vi "UI Laser Page.vi"(8 "error in":errorcluster) -> (0 "error out":errorcluster)   [LabVIEW 2019, in "UIs.lvlib"]
uses:
  UIs.lvlib
  <vilib>/Utility/miscctls.llb/LVPointTypeDef.ctl
  Camera/Andor/Andor.lvlib
  Laser/Coherent/Coherent.lvlib
  Motion/Allmotion/Allmotion.lvlib
  Image/Image.lvlib
  Controller/Controller.lvlib
  Initialize/Initialize.lvlib
panel:
  in  "Align Laser":bool
  in  "Search Focus":bool
  in  "Back":bool
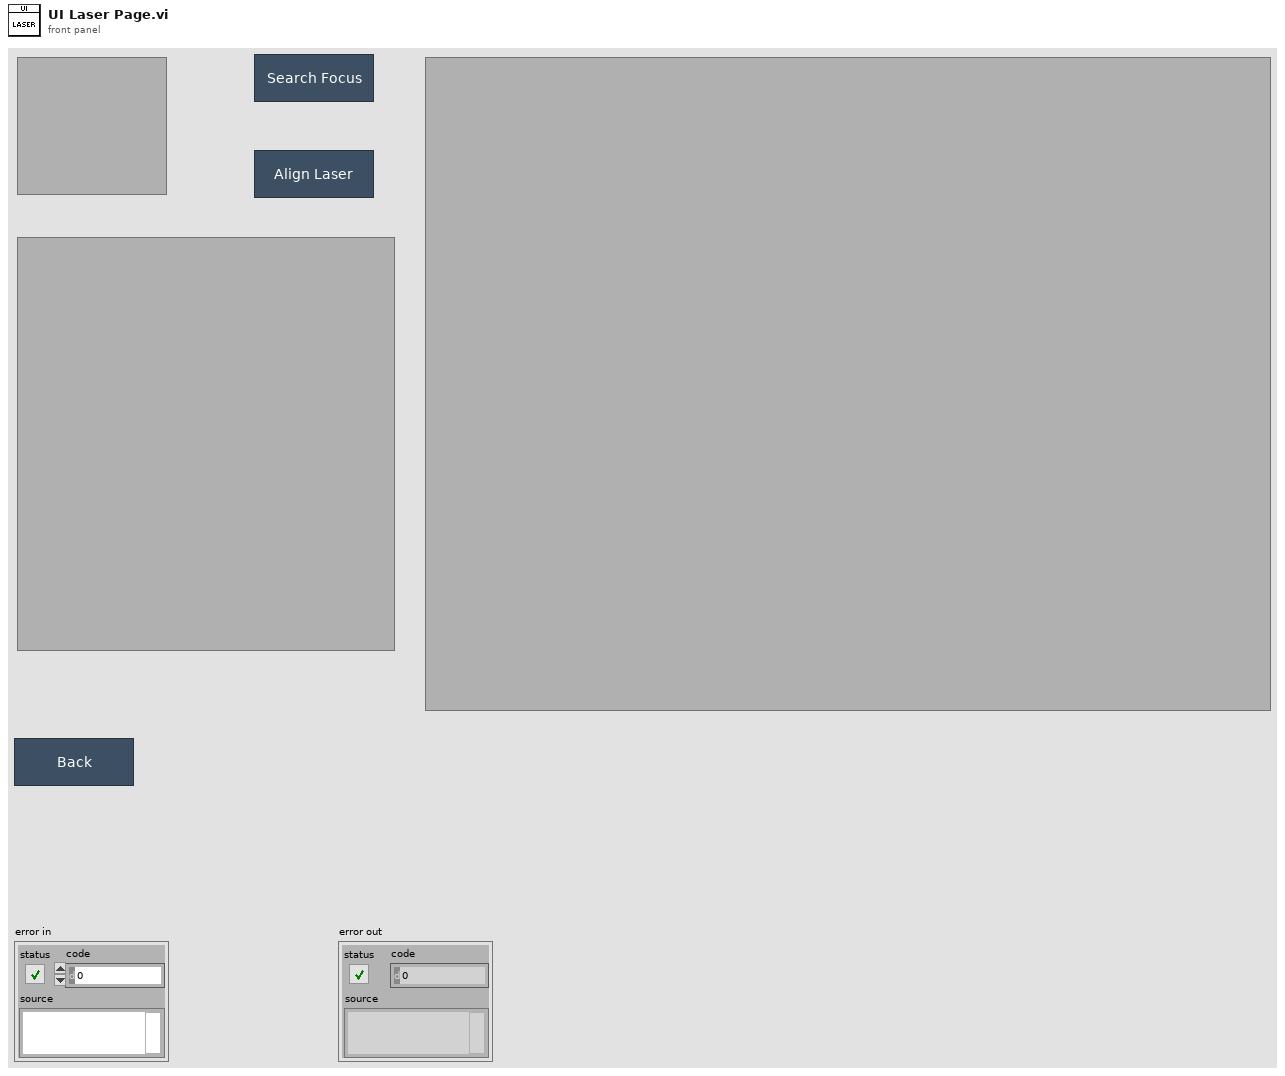
[diagram p1: front panel]
types:
  T1 = typedef "LVPointTypeDef.ctl" = cluster{"Horizontal":i16, "Vertical":i16}
  T2 = typedef "Allmotion.lvlib/SEQ Data.ctl" = cluster{"Position":i32[], "Arrived?":bool, "VISA name":refnum<visa-resource-name>, "Initialize Done?":bool, "State":string, "VI Refnum":refnum<vi>, "Dichroic Position":string[]}
  T3 = typedef "Andor.lvlib/SEQ Data.ctl" = cluster{"Initialize Sucess?":bool, "Image Ref":T4, "VI Refnum":refnum<vi>}
  T4 = typedef "IMAQ Image.ctl" = refnum<image>
  T5 = typedef "Coherent.lvlib/SEQ Data.ctl" = cluster{"Initialize Success?":bool, "VI Refnum":refnum<vi>}
  T6 = typedef "Initialize.lvlib/SEQ Data.ctl" = cluster{"Folder Path":path}
  T7 = typedef "Image.lvlib/SEQ Data.ctl" = cluster{"Acquire Done?":bool, "Focus Done?":bool, "Align Done?":bool, "No Position Match?":bool, "Best Wheel Position":string, "Match Done?":bool, "Match Score":dbl, "Focus Score":dbl, "Match Position":cluster{"x":sgl, "y":sgl}, "Flower Position":i32[]}
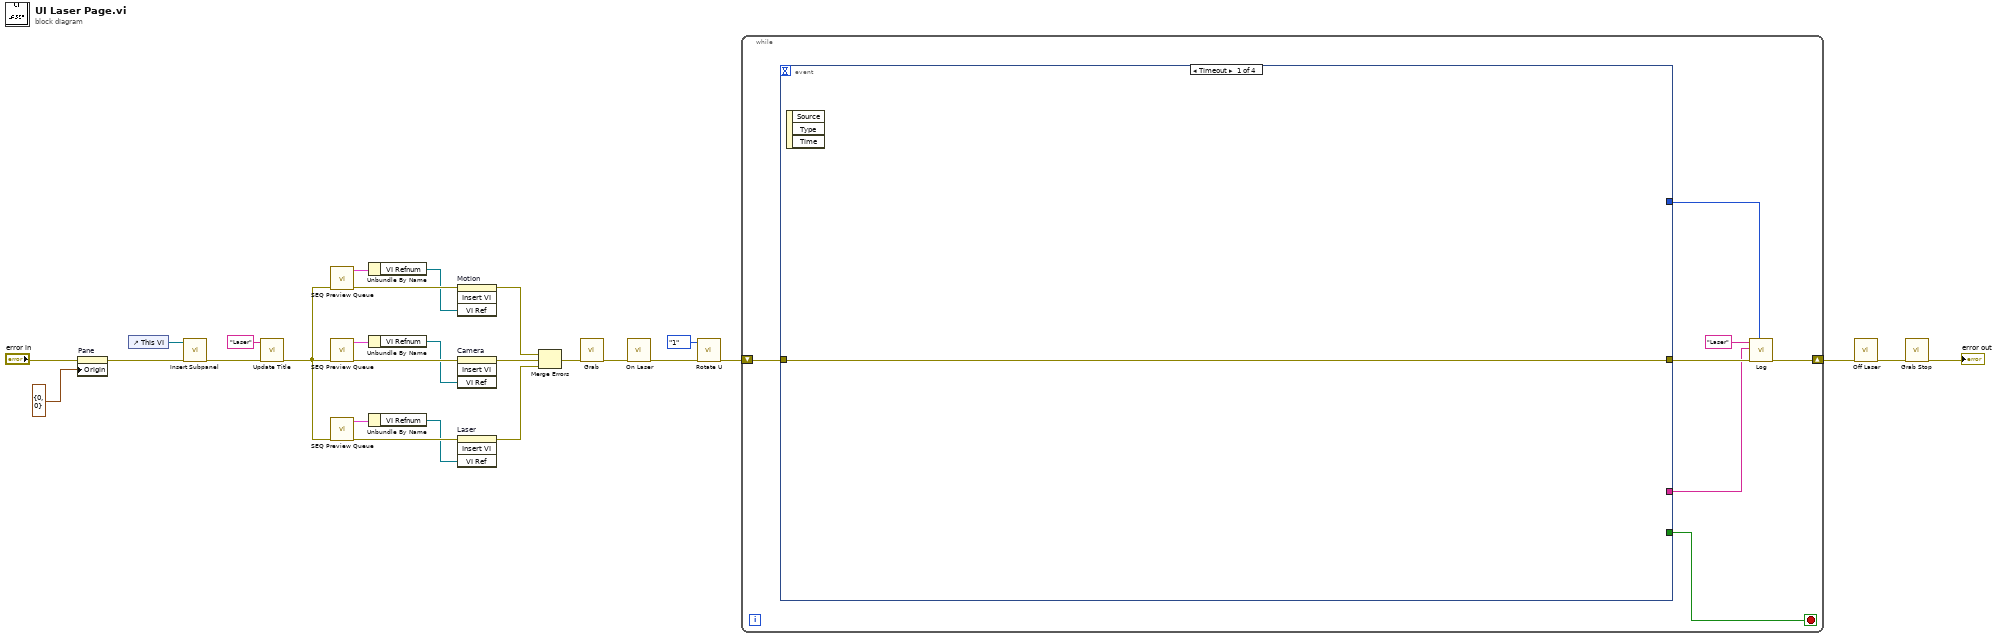
[diagram p0: block diagram]
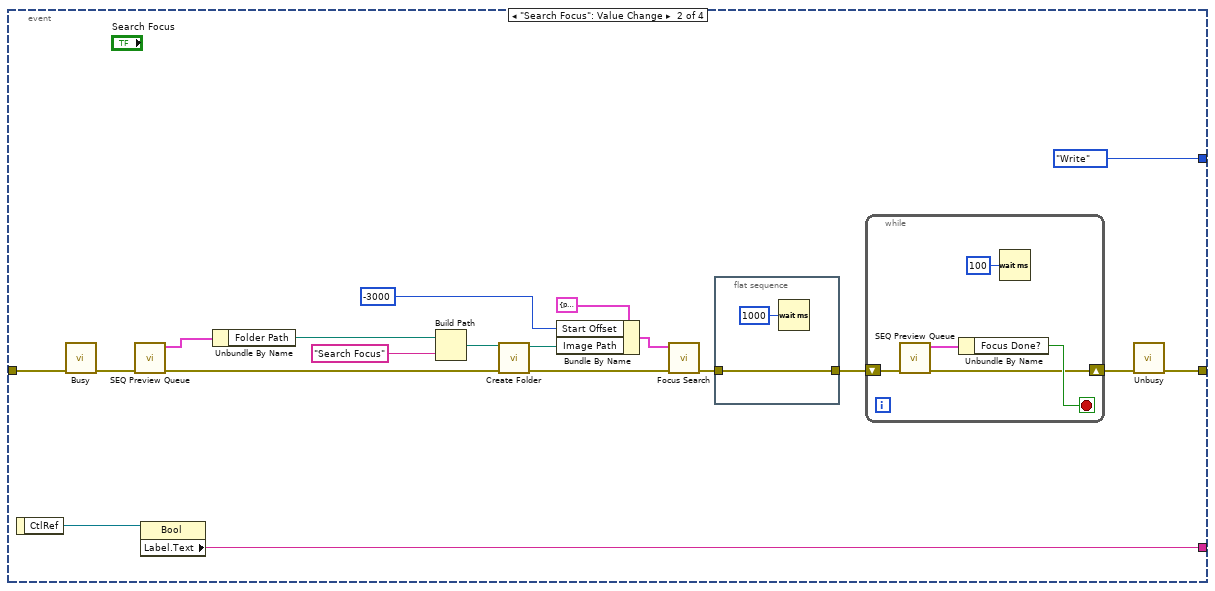
[diagram p2: hidden frame]
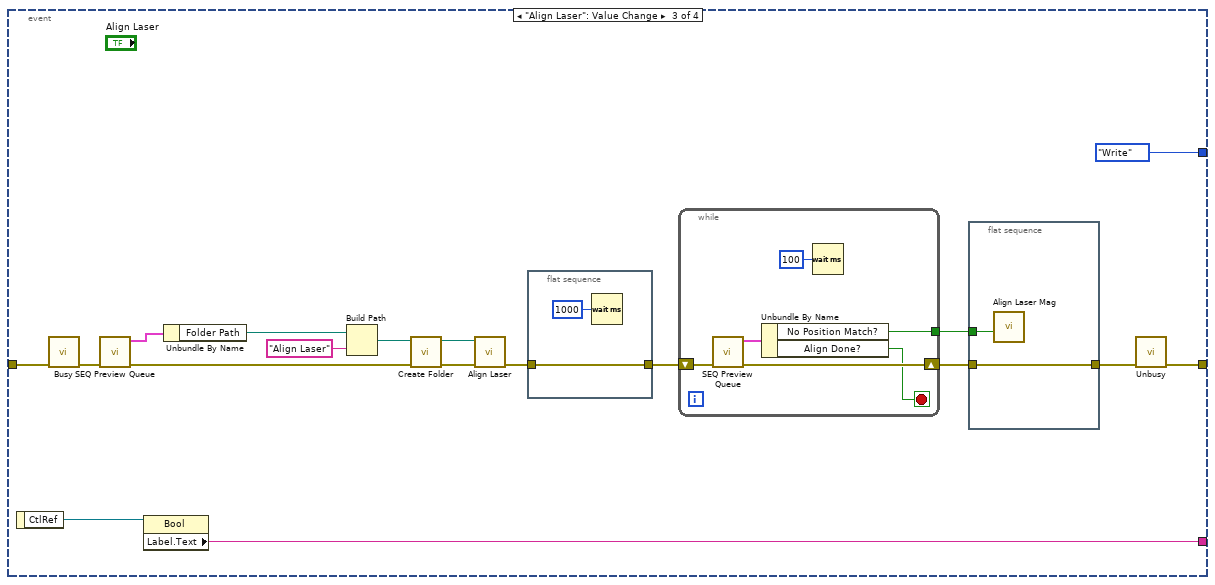
[diagram p3: hidden frame]
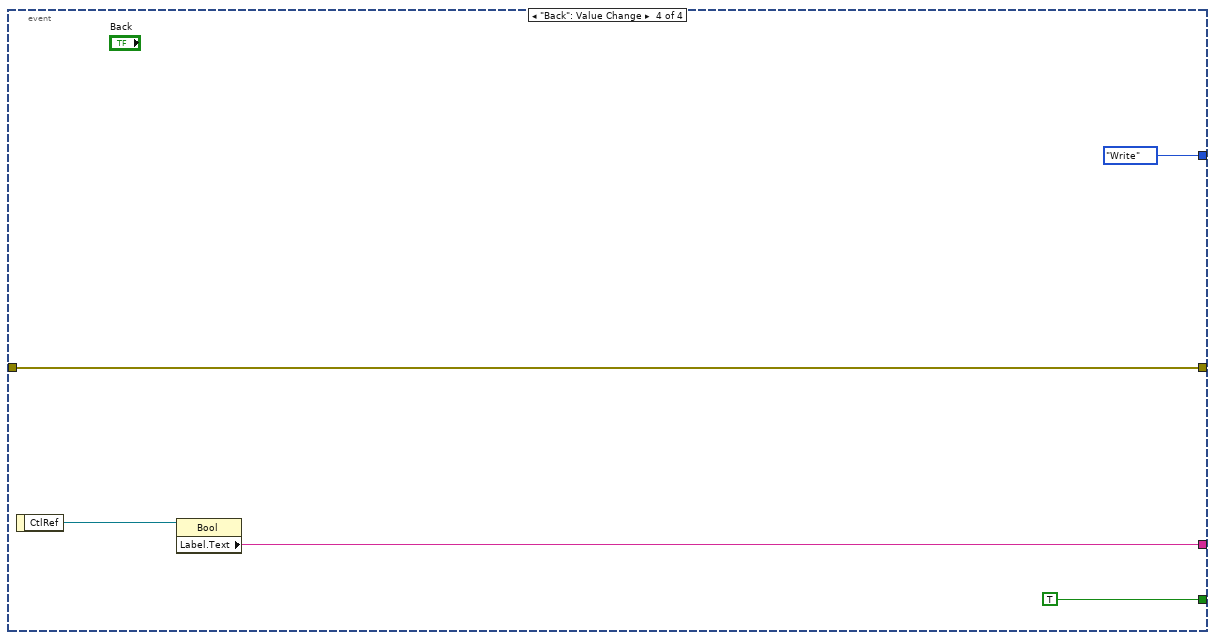
[diagram p4: hidden frame]
diagram:
  n1 = property on="Pane" class="Pane"(error in="error in", "Origin"=T1 {"Horizontal"=0, "Vertical"=0}) -> (error out=w14:errorcluster)  [unwired: 1 in, 1 out]
  n2 = control-ref of="This VI"() -> (w4:refnum<vi>)
  n3 = call "Insert Subpanel.vi"("Error In"=w14, "VI Refnum"=w4) -> ("Error Out"=w3:errorcluster)  [unwired: 9 in]
  n4 = call "Update Title.vi"("Error In"=w3, "Title"="Laser") -> ("Error Out"=w2:errorcluster)  [unwired: 9 in]
  n5 = call "SEQ Preview Queue.vi"("error in"=w2) -> ("error out"=w24:errorcluster, "SEQ Data"=w23:T2)  [unwired: 9 in]
  n6 = call "SEQ Preview Queue.vi"("error in"=w2) -> ("error out"=w26:errorcluster, "SEQ Data"=w27:T3)  [unwired: 9 in]
  n7 = call "SEQ Preview Queue.vi"("error in"=w2) -> ("error out"=w22:errorcluster, "SEQ Data"=w21:T5)  [unwired: 9 in]
  n8 = Unbundle By Name(w23) -> ("VI Refnum"=w20:refnum<vi>)
  n9 = Unbundle By Name(w27) -> ("VI Refnum"=w25:refnum<vi>)
  n10 = Unbundle By Name(w21) -> ("VI Refnum"=w19:refnum<vi>)
  n11 = invoke on="Motion" class="SubPnl" method="Insert VI"(error in=w24, "VI Ref"=w20) -> (error out=w18:errorcluster)  [unwired: 2 in, 3 out]
  n12 = invoke on="Camera" class="SubPnl" method="Insert VI"(error in=w26, "VI Ref"=w25) -> (error out=w17:errorcluster)  [unwired: 2 in, 3 out]
  n13 = invoke on="Laser" class="SubPnl" method="Insert VI"(error in=w22, "VI Ref"=w19) -> (error out=w16:errorcluster)  [unwired: 2 in, 3 out]
  n14 = Merge Errors(w18, w17, w16) -> (w12:errorcluster)
  n15 = call "Grab.vi"("Error In"=w12) -> ("Error Out"=w10:errorcluster)  [unwired: 10 in]
  n16 = call "On Laser.vi"("Error In"=w10) -> ("Error Out"=w7:errorcluster)  [unwired: 10 in]
  n17 = call "Rotate U.vi"("Error In"=w7, "Cube"=enum16{"1", "2", "3", "4", "5", "6", "7", "8"}."1") -> ("Error Out"=w6:errorcluster)  [unwired: 9 in]
  n18 = while {
    shift-right: [w31] -> w9
    shift-left: w6 -> [w34]
    stop <- w33 stop-if-true
    n19 = event shown="[0] Timeout" {
      selector: _ -> [_ _ _ _]
      dyn-events: _ -> [_ _ _ _]
      timeout: _ -> [_ _ _ _]
      tunnel: w34 -> [w35 w42 w68 w94]
      tunnel: [w35 w39 w65 w94] -> w32
      tunnel: [_ _ _ TRUE] -> w33
      tunnel: [_ w37 w63 w91] -> w29
      tunnel: [_ enum16{"None", "Write"}."Write" ("Action") enum16{"None", "Write"}."Write" ("Action") enum16{"None", "Write"}."Write" ("Action")] -> w28
      event Timeout {
        n20 = event-data() -> ()  [unwired: 1 in, 3 out]
      }
      event "Search Focus": Value Change {
        n21 = event-data() -> ("CtlRef"=w38:refnum<vi>)  [unwired: 1 in]
        n22 = call "Busy.vi"("Error In"=w42) -> ("Error Out"=w41:errorcluster)  [unwired: 10 in]
        n23 = call "SEQ Preview Queue.vi"("error in"=w41) -> ("error out"=w45:errorcluster, "SEQ Data"=w44:T6)  [unwired: 9 in]
        n24 = property class="Bool"(reference=w38) -> ("Label.Text"=w37:string)  [unwired: 1 in, 2 out]
        n25 = Unbundle By Name(w44) -> ("Folder Path"=w43:path)
        n26 = Build Path(base path=w43, name or relative path="Search Focus") -> (appended path=w48:path)
        n27 = call "Create Folder.vi"("error in"=w45, "Path in"=w48) -> ("error out"=w47:errorcluster, "Path out"=w46:path)  [unwired: 8 in]
        n28 = Bundle By Name(cluster=cluster{"Image Path":path, "Start Offset":i32} {"Image Path"=path "", "Start Offset"=0} ("Focus Data"), "Start Offset"=-3000, "Image Path"=w46) -> (w51:cluster{"Image Path":path, "Start Offset":i32})
        n29 = call "Focus Search.vi"("Error In"=w47, "Focus Data"=w51) -> ("Error Out"=w54:errorcluster)  [unwired: 9 in]
        n30 = flat-sequence {
          tunnel: w54 -> [w60]
          tunnel: [w60] -> w53
          frame #0 {
            n31 = Wait (ms)(milliseconds to wait=u32 1000) -> ()  [unwired: 1 out]
          }
        }
        n32 = while {
          shift-right: [w55] -> w40
          shift-left: w53 -> [w59]
          stop <- w56 stop-if-true
          n33 = call "SEQ Preview Queue.vi"("error in"=w59) -> ("error out"=w55:errorcluster, "SEQ Data"=w57:T7)  [unwired: 9 in]
          n34 = Unbundle By Name(w57) -> ("Focus Done?"=w56:bool)
          n35 = Wait (ms)(milliseconds to wait=u32 100) -> ()  [unwired: 1 out]
        }
        n36 = call "Unbusy.vi"("Error In"=w40) -> ("Error Out"=w39:errorcluster)  [unwired: 10 in]
      }
      event "Align Laser": Value Change {
        n37 = event-data() -> ("CtlRef"=w64:refnum<vi>)  [unwired: 1 in]
        n38 = call "Busy.vi"("Error In"=w68) -> ("Error Out"=w67:errorcluster)  [unwired: 10 in]
        n39 = call "SEQ Preview Queue.vi"("error in"=w67) -> ("error out"=w69:errorcluster, "SEQ Data"=w71:T6)  [unwired: 9 in]
        n40 = property class="Bool"(reference=w64) -> ("Label.Text"=w63:string)  [unwired: 1 in, 2 out]
        n41 = Unbundle By Name(w71) -> ("Folder Path"=w70:path)
        n42 = Build Path(base path=w70, name or relative path="Align Laser") -> (appended path=w73:path)
        n43 = call "Create Folder.vi"("error in"=w69, "Path in"=w73) -> ("error out"=w74:errorcluster, "Path out"=w72:path)  [unwired: 8 in]
        n44 = call "Align Laser.vi"("Error In"=w74, "Image Path"=w72) -> ("Error Out"=w79:errorcluster)  [unwired: 9 in]
        n45 = flat-sequence {
          tunnel: w79 -> [w88]
          tunnel: [w88] -> w78
          frame #0 {
            n46 = Wait (ms)(milliseconds to wait=u32 1000) -> ()  [unwired: 1 out]
          }
        }
        n47 = while {
          shift-right: [w84] -> w76
          shift-left: w78 -> [w87]
          tunnel: [w82] -> w77
          stop <- w83 stop-if-true
          n48 = call "SEQ Preview Queue.vi"("error in"=w87) -> ("error out"=w84:errorcluster, "SEQ Data"=w85:T7)  [unwired: 9 in]
          n49 = Unbundle By Name(w85) -> ("No Position Match?"=w82:bool, "Align Done?"=w83:bool)
          n50 = Wait (ms)(milliseconds to wait=u32 100) -> ()  [unwired: 1 out]
        }
        n51 = flat-sequence {
          tunnel: w77 -> [w81]
          tunnel: w76 -> [w80]
          tunnel: [w80] -> w66
          frame #0 {
            n52 = call "Align Laser Mag"("Enable"=w81) -> ()  [unwired: 9 in, 2 out]
          }
        }
        n53 = call "Unbusy.vi"("Error In"=w66) -> ("Error Out"=w65:errorcluster)  [unwired: 10 in]
      }
      event "Back": Value Change {
        n54 = event-data() -> ("CtlRef"=w92:refnum<vi>)  [unwired: 1 in]
        n55 = property class="Bool"(reference=w92) -> ("Label.Text"=w91:string)  [unwired: 1 in, 2 out]
      }
    }
    n56 = call "Log.vi"("Action"=w28, "error in"=w32, "State"=w29, "Page Name"="Laser") -> ("error out"=w31:errorcluster)  [unwired: 7 in]
  }
  n57 = call "Off Laser.vi"("Error In"=w9) -> ("Error Out"=w8:errorcluster)  [unwired: 10 in]
  n58 = call "Grab Stop.vi"("Error In"=w8) -> ("Error Out"=→"error out":errorcluster)  [unwired: 10 in]
